vi "Highlight Out of Tolerances.vi"(0 "TableRef":refnum<vi>, 7 "Array":string[][](array[string])) -> ()   [LabVIEW 2019]
uses:
  <vilib>/Utility/miscctls.llb/LVRowAndColumnTypeDef.ctl
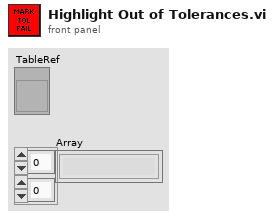
[diagram p1: front panel]
types:
  T1 = typedef "LVRowAndColumnTypeDef.ctl" = cluster{"Row":i32, "Column":i32}
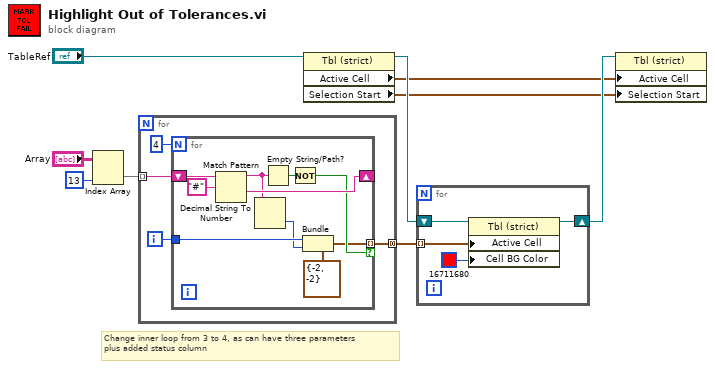
[diagram p0: block diagram]
diagram:
  # "Change inner loop from 3 to 4, as can have three parameters\nplus added status column"
  n1 = Index Array(array="Array", index (col)=13 ("disabled index (col)")) -> (element=w7:string[])  [unwired: 1 in]
  n2 = for {
    tunnel: w7 -> [w13] mode=indexing
    tunnel: [w10] -> w6 mode=concatenating
    i -> [w11]
    n3 = for {
      N: 4 -> [_]
      shift-right: [w22] -> _
      shift-left: w13 -> [w23]
      tunnel: [w14] -> w10 mode=indexing if=w18
      tunnel: w11 -> [w16]
      n4 = Match Pattern(string=w23, regular expression="#") -> (before substring=w20:string, after substring=w22:string)  [unwired: 1 in, 2 out]
      n5 = Decimal String To Number(string=w20) -> (number=w15:i32)  [unwired: 2 in, 1 out]
      n6 = Empty String/Path?(string/path=w20) -> (empty?=w19:bool)
      n7 = Not(x=w19) -> (.not. x?=w18:bool)
      n8 = Bundle(cluster=T1 {"Row"=-2, "Column"=-2} ("Active Cell:Active Cell"), "Row"=w16, "Column"=w15) -> (w14:T1)
    }
  }
  n9 = property on="Property Node" class="Tbl (strict)"(reference="TableRef") -> (reference out=w5:refnum<vi>, "Active Cell"=w3:T1, "Selection Start"=w2:T1)  [unwired: 1 in, 1 out]
  n10 = for {
    tunnel: w6 -> [w27] mode=indexing
    shift-right: [w25] -> w4
    shift-left: w5 -> [w24]
    n11 = property on="Property Node" class="Tbl (strict)"(reference=w24, "Active Cell"=w27, "Cell BG Color"=u32 16711680) -> (reference out=w25:refnum<vi>)  [unwired: 1 in, 1 out]
  }
  n12 = property on="Property Node" class="Tbl (strict)"(reference=w4, "Active Cell"=w3, "Selection Start"=w2) -> ()  [unwired: 1 in, 2 out]
